vi "Centrifuge Init Selection.vi"(8 "error in (no error)":errorcluster, 11 "Pump Settings In":T1={"Output Device"=enum."Default", "EPOS4 Settings"={"VISA resource name"="", "axis"={"keyHandle"=1, "nodeId"=1}, "Simulated?"=FALSE}}) -> (0 "error out":errorcluster, 2 "Initialized":bool, 3 "Pump Settings Out":T1={"Output Device"=enum."Default", "EPOS4 Settings"={"VISA resource name"="", "axis"={"keyHandle"=1, "nodeId"=1}, "Simulated?"=FALSE}})   [LabVIEW 2018, in "Centrifuge Module.lvlib" / "Centrifuge Module Engine.lvlib"]
uses:
  Centrifuge Module Engine.lvlib
  Centrifuge Settings Cluster.ctl
  EPOS4/Controls/Device Selection.ctl
  EPOS4/Controls/EPOS Communication Settings.ctl
  Centrifuge Module.lvlib
  EPOS4/EPOS4.lvlib
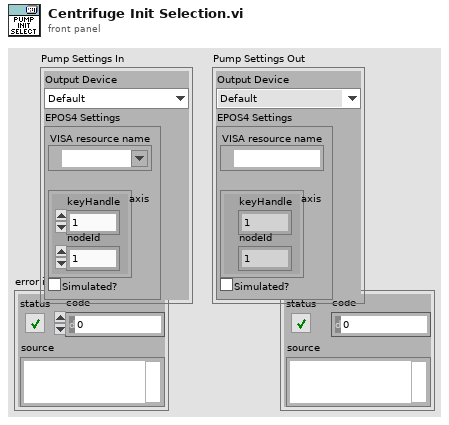
[diagram p1: front panel]
types:
  T1 = typedef "Centrifuge Module.lvlib/Centrifuge Settings Cluster.ctl" = cluster{"Output Device":T2, "EPOS4 Settings":T3}
  T2 = typedef "Device Selection.ctl" = enum16{"Default", "EPOS4"}
  T3 = typedef "EPOS4.lvlib/EPOS Communication Settings.ctl" = cluster{"VISA resource name":refnum<visa-resource-name>, "axis":cluster{"keyHandle":u32, "nodeId":u16}, "Simulated?":bool}
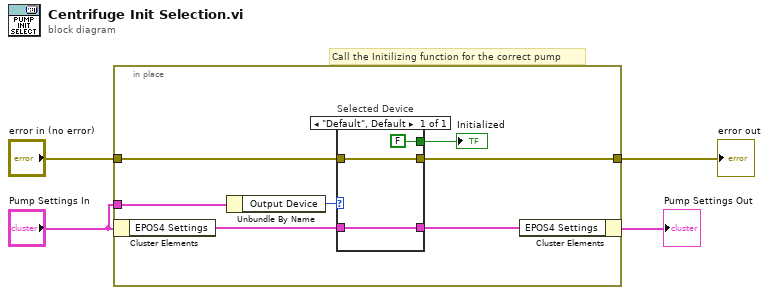
[diagram p0: block diagram]
diagram:
  # "Call the Initilizing function for the correct pump"
  n1 = in-place {
    in-place-border: [w9] -> w4
    in-place-border: "error in (no error)" -> [w8]
    in-place-border: "Pump Settings In" -> [w7]
    n2 = in-place-cluster #1("Pump Settings In") -> ("EPOS4 Settings"=w6:T3)
    n3 = Unbundle By Name(w7) -> ("Output Device"=w10:T2)
    n4 = case "Selected Device" shown="\"Default\", Default" w10 {
      tunnel: w6 -> [w14]
      tunnel: [w14] -> w5
      tunnel: w8 -> [w13]
      tunnel: [w13] -> w9
      tunnel: [FALSE ("Initialized")] -> w11
      frame "Default", Default {
      }
    }
    "Initialized" <- w11
    n5 = in-place-cluster #1("EPOS4 Settings"=w5) -> (→"Pump Settings Out":T1)
  }
  "error out" <- w4
